vi "set_frame_rate.vi"(8 "error in (no error)":errorcluster, 10 "frame rate":dbl[unit], 11 "MG090622IMAQCamera.lvclass in":refnum<class "DAQ_MG090622Camera.lvclass">) -> (0 "error out":errorcluster, 3 "MG090622IMAQCamera.lvclass out":refnum<class "DAQ_MG090622Camera.lvclass">)   [LabVIEW 2010]
uses:
  DAQ_MG090622Camera.lvclass
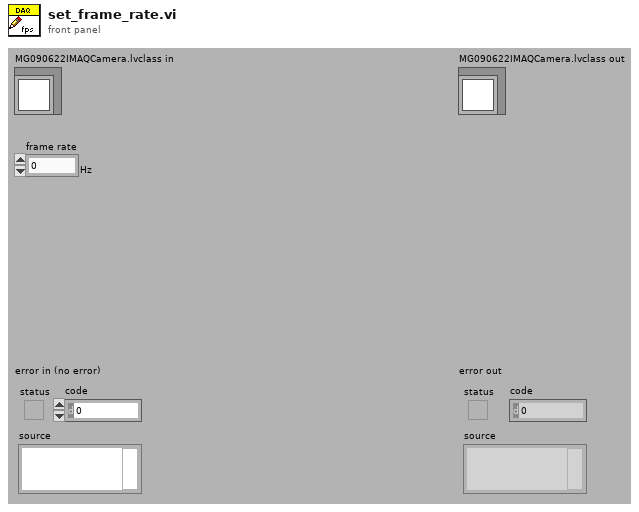
[diagram p1: front panel]
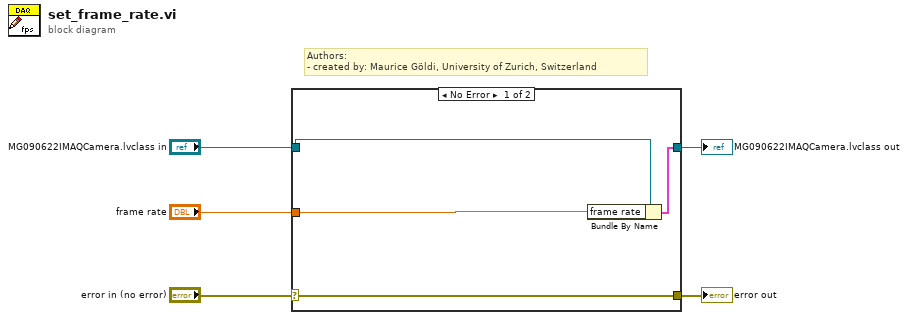
[diagram p0: block diagram]
diagram:
  # "Authors: \n- created by: Maurice Göldi, University of Zurich, Switzerland"
  n1 = case shown="No Error" "error in (no error)" {
    selector: "error in (no error)" -> [w9 w10]
    tunnel: [w9 w10] -> w4
    tunnel: [w7 w11] -> w2
    tunnel: "MG090622IMAQCamera.lvclass in" -> [w8 w11]
    tunnel: "frame rate" -> [w6 _]
    frame No Error {
      n2 = Bundle By Name(cluster=w8, "frame rate"=w6) -> (w7:cluster{})
    }
    frame Error {
    }
  }
  "error out" <- w4
  "MG090622IMAQCamera.lvclass out" <- w2
